vi "GetCoeffsAndComp.vi"(10 "mutedData":dbl[](array[numeric])) -> (2 "boostedData":dbl[](array[numeric]))   [LabVIEW 2011]
uses:
  Globals/Meas_global.vi
  Globals/Constants_global.vi
panel:
  out "TubingCorrectionFile (pre-set!)":path
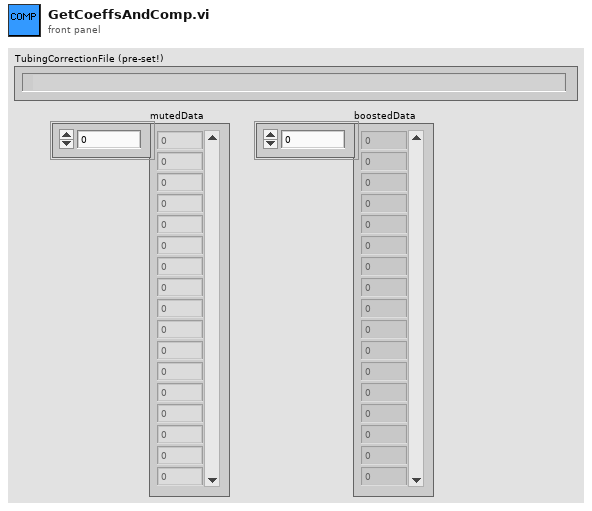
[diagram p1: front panel]
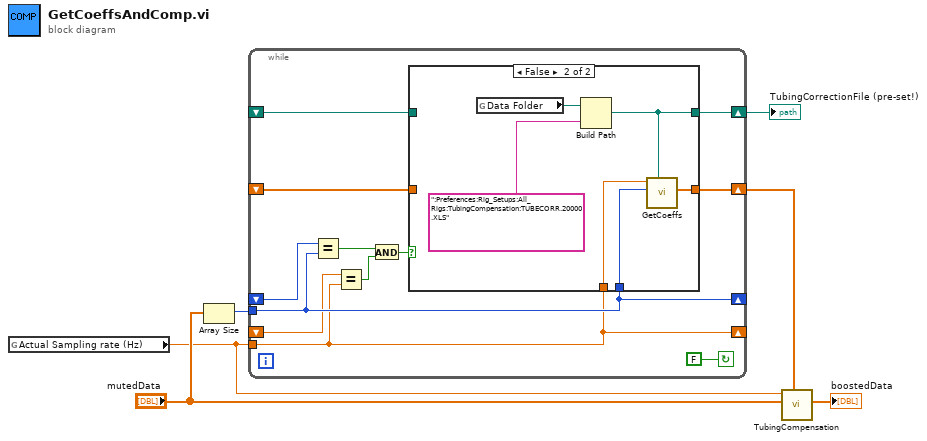
[diagram p0: block diagram]
diagram:
  n1 = global read "Meas_global.vi" "Actual Sampling rate (Hz)"() -> (w3:dbl)
  n2 = Array Size(array="mutedData") -> (size(s)=w5:i32)
  n3 = while {
    shift-right: [w17] -> w2
    shift-left: _ -> [w18]
    shift-right: [w14] -> _
    shift-left: _ -> [w15]
    shift-right: [w12] -> _
    shift-left: _ -> [w13]
    tunnel: w5 -> [w14]
    tunnel: w3 -> [w12]
    shift-right: [w8] -> w1
    shift-left: _ -> [w7]
    stop <- FALSE continue-if-true
    n4 = Equal?(x=w15, y=w14) -> (x = y?=w9:bool)
    n5 = Equal?(x=w13, y=w12) -> (x = y?=w10:bool)
    n6 = And(x=w9, y=w10) -> (x .and. y?=w11:bool)
    n7 = case shown="False" w11 {
      tunnel: [w20 w26] -> w17
      tunnel: w18 -> [w20 _]
      tunnel: w12 -> [_ w25]
      tunnel: w14 -> [_ w22]
      tunnel: [w19 w21] -> w8
      tunnel: w7 -> [w19 _]
      frame True {
      }
      frame False {
        n8 = global read "Constants_global.vi" "Data Folder"() -> (w24:path)
        n9 = Build Path(base path=w24, name or relative path=":Preferences:Rig_Setups:All_Rigs:TubingCompensation:TUBECORR.20000.XLS") -> (appended path=w21:path)
        n10 = call "GetCoeffs.vi"("PathToFile"=w21, "SignalLength"=w22, "fs (Hz)"=w25) -> ("NyquistLimitedCoefficients"=w26:dbl[])  [unwired: 8 in]
      }
    }
  }
  "TubingCorrectionFile (pre-set!)" <- w1
  n11 = call "TubingCompensation.vi"("NyquistLimitedCoefficients"=w2, "mutedData"="mutedData", "SamplingFreq"=w3) -> ("boostedData"=→"boostedData":dbl[])  [unwired: 8 in]
